vi "Post action control PPMS2.vi"(1 "Action":u16(ring)=4 items=["Check Temperature", "Check Field Value", "Check Position", "Wait", "Do Nothing"], 2 "Scan Parameters":T1={"DAQ Channel"=3, "Label"="\nappliedVsg2=", "Scaled low"=-0.11, "Scaled high"=0.31, "Start"=-0.01, "End"=0.4, "Step"=0.01, "Scale?"=FALSE} {"Step" format="%#_6p"; "End" format="%#_6p"; "Start" format="%#_6p"; "Scaled high" format="%#_6p"; "Scaled low" format="%#_6p"}, 3 "Index":i32=41) -> ()   [LabVIEW 2013]
uses:
  PPMS Global.vi
panel:
  in  "milliseconds to wait":u32=10000
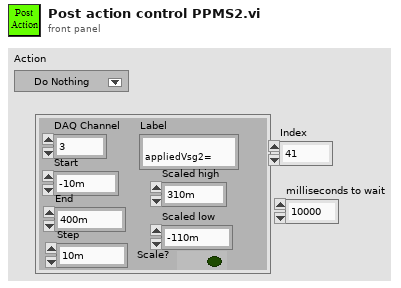
[diagram p1: front panel]
types:
  T1 = cluster{"DAQ Channel":i32, "Label":string, "Scaled low":dbl, "Scaled high":dbl, "Start":dbl, "End":dbl, "Step":dbl, "Scale?":bool}
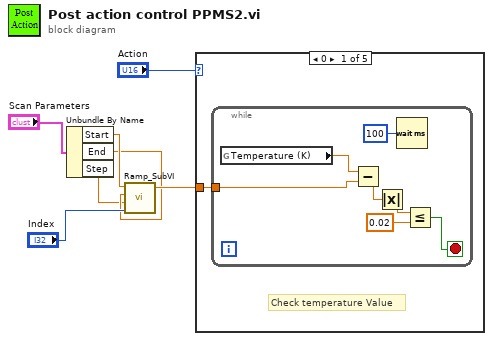
[diagram p0: block diagram]
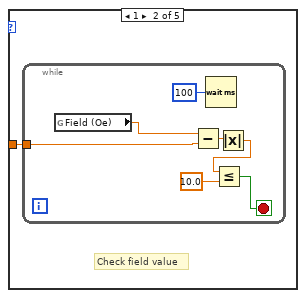
[diagram p2: hidden frame]
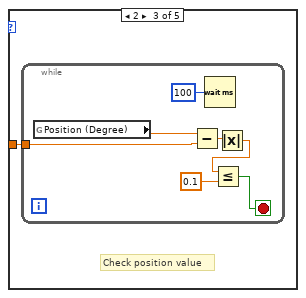
[diagram p3: hidden frame]
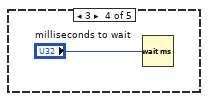
[diagram p4: hidden frame]
diagram:
  n1 = Unbundle By Name("Scan Parameters") -> ("Start"=w4:dbl, "End"=w3:dbl, "Step"=w2:dbl)
  n2 = call <userlib>:"Ramp_SubVI.vi"("index"="Index", "step"=w2, "end"=w3, "start"=w4) -> ("Numeric"=w6:dbl)  [unwired: 1 in, 1 out]
  n3 = case shown="0" "Action" {
    tunnel: w6 -> [w8 w16 w24 _ _]
    frame 0 {
      # "Check temperature Value"
      n4 = while {
        tunnel: w8 -> [w11]
        stop <- w9 stop-if-true
        n5 = global read "PPMS Global.vi" "Temperature (K)"() -> (w10:dbl)
        n6 = Subtract(x=w10, y=w11) -> (x-y=w15:dbl)
        n7 = Absolute Value(x=w15) -> (abs(x)=w14:dbl)
        n8 = Wait (ms)(milliseconds to wait=u32 100) -> ()  [unwired: 1 out]
        n9 = Less Or Equal?(x=w14, y=0.02) -> (x <= y?=w9:bool)
      }
    }
    frame 1 {
      # "Check field value"
      n10 = while {
        tunnel: w16 -> [w23]
        stop <- w19 stop-if-true
        n11 = global read "PPMS Global.vi" "Field (Oe)"() -> (w17:dbl)
        n12 = Subtract(x=w17, y=w23) -> (x-y=w22:dbl)
        n13 = Wait (ms)(milliseconds to wait=u32 100) -> ()  [unwired: 1 out]
        n14 = Absolute Value(x=w22) -> (abs(x)=w21:dbl)
        n15 = Less Or Equal?(x=w21, y=10.0) -> (x <= y?=w19:bool)
      }
    }
    frame 2 {
      # "Check position value"
      n16 = while {
        tunnel: w24 -> [w31]
        stop <- w27 stop-if-true
        n17 = global read "PPMS Global.vi" "Position (Degree)"() -> (w25:dbl)
        n18 = Subtract(x=w25, y=w31) -> (x-y=w30:dbl)
        n19 = Wait (ms)(milliseconds to wait=u32 100) -> ()  [unwired: 1 out]
        n20 = Absolute Value(x=w30) -> (abs(x)=w29:dbl)
        n21 = Less Or Equal?(x=w29, y=0.1) -> (x <= y?=w27:bool)
      }
    }
    frame 3 {
      n22 = Wait (ms)(milliseconds to wait="milliseconds to wait") -> ()  [unwired: 1 out]
    }
    frame 4, Default {
      # "Do nothing"
    }
  }
